vi "pll-read.vi"(8 "error in (no error)":errorcluster, 11 "PLL reader.lvclass":refnum<class "PLL reader.lvclass">) -> (0 "error out":errorcluster, 2 "Result":dbl[](array[numeric]), 3 "PLL reader.lvclass Out":refnum<class "PLL reader.lvclass">)   [LabVIEW 2018, in "PLL reader.lvclass"]
uses:
  PLL reader.lvclass
  Users/Shared/github/NHMFL_Core/Libraries/Instruments/Instrument Driver/Instrument Driver.lvclass
  resonant_ultrasound_arxiv/maglab ultrasound -- arkady --arxiv/publisher action.ctl
  NHMFL_Core/Libraries/Instruments/Instrument Driver/Instrument Driver.lvclass/Instrument Driver.ctl
  NHMFL_Core/Libraries/Instruments/Instrument Driver/Write Channel names.vi
  NHMFL_Core/Libraries/Instruments/Instrument Driver/Write Channel units.vi
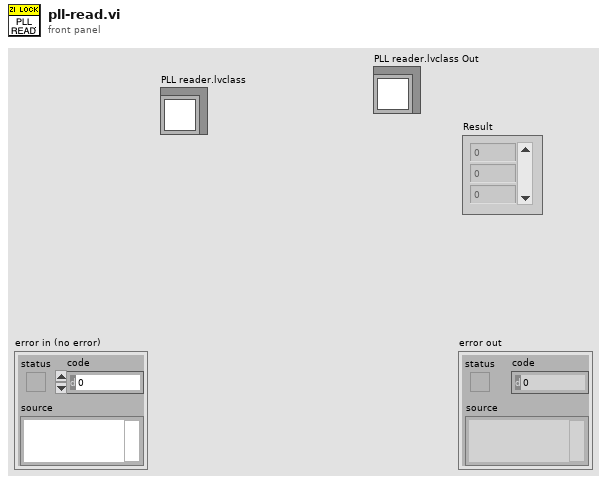
[diagram p1: front panel]
types:
  T1 = typedef "publisher action.ctl" = enum16{"set", "get"}
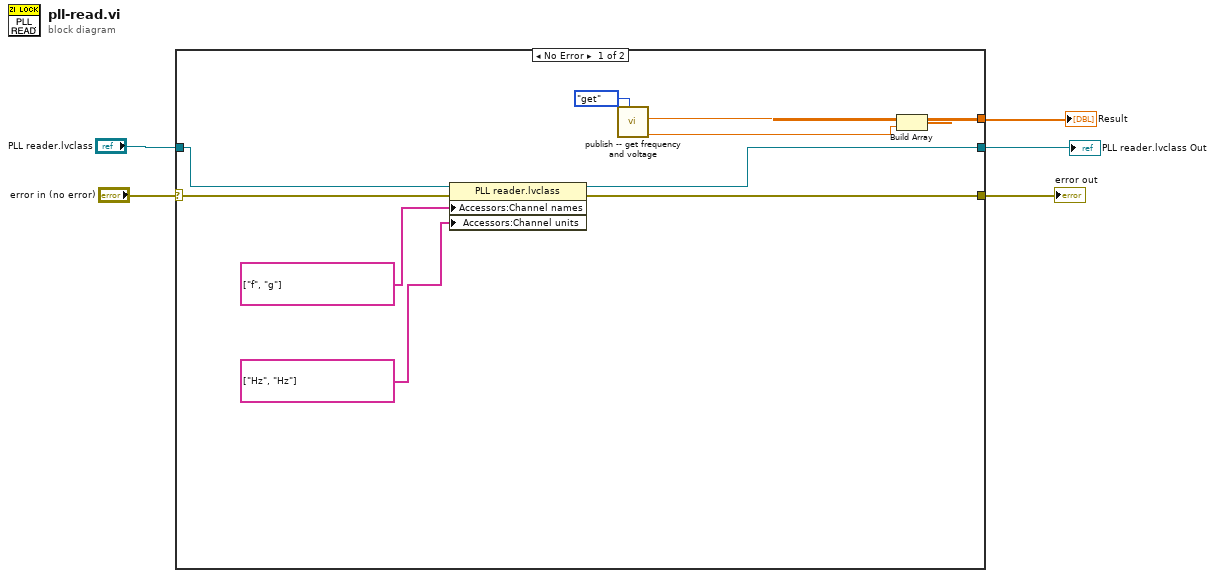
[diagram p0: block diagram]
diagram:
  n1 = case shown="No Error" "error in (no error)" {
    selector: "error in (no error)" -> [w12 w17]
    tunnel: [w11 w17] -> w4
    tunnel: [w13 w16] -> w2
    tunnel: "PLL reader.lvclass" -> [w14 w16]
    tunnel: [w15 _] -> w3
    frame No Error {
      n2 = property class="PLL reader.lvclass"(reference=w14, error in=w12, "Accessors:Channel names"=string[] ["f", "g"] ("Channel names"), "Accessors:Channel units"=string[] ["Hz", "Hz"] ("Channel names")) -> (reference out=w13:refnum<class "PLL reader.lvclass">, error out=w11:errorcluster)
      n3 = call "publish -- get frequency and voltage.vi"("publisher action"=publisher_action."get") -> ("gamma OUT (Hz)"=w6:dbl, "freq out (Hz)"=w7:dbl)  [unwired: 8 in, 1 out]
      n4 = Build Array(w7, w6) -> (w15:dbl[])
    }
    frame Error {
    }
  }
  "error out" <- w4
  "Result" <- w3
  "PLL reader.lvclass Out" <- w2
